vi "connect.vi"(0 "username":string="user", 1 "schema":string="public", 5 "password":string="password", 7 "host":string="localhost", 9 "port":i32=33060, 11 "error in (no error)":errorcluster) -> (4 "DB Session ID":i32, 15 "error out":errorcluster)   [LabVIEW 2022 SP3, in "Database.lvlib"]
uses:
  Database.lvlib
  bin/Database.dll
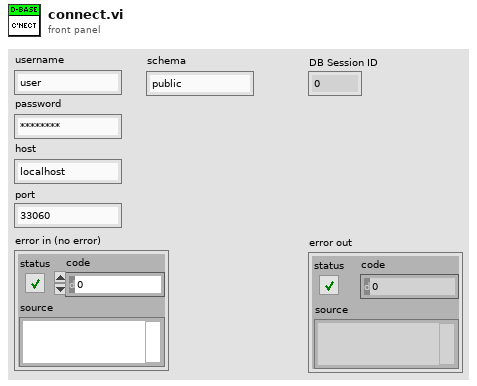
[diagram p1: front panel]
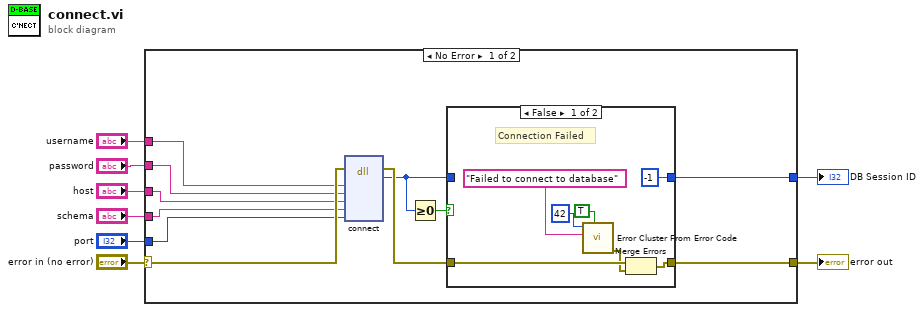
[diagram p0: block diagram]
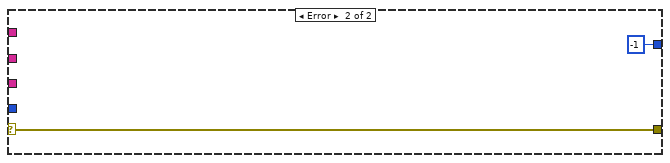
[diagram p3: hidden frame]
diagram:
  n1 = case shown="No Error" "error in (no error)" {
    selector: "error in (no error)" -> [w19 w30]
    tunnel: [w15 w30] -> w7
    tunnel: "username" -> [w13 _]
    tunnel: "password" -> [w12 _]
    tunnel: "host" -> [w11 _]
    tunnel: "port" -> [w10 _]
    tunnel: [w14 -1 ("return type")] -> w2
    tunnel: "schema" -> [w9 _]
    frame No Error {
      n2 = dll-call lib="C:/Users/Caleb/Desktop/nebraska-silicon-lab/pixel-gantry-control/Gantry/Shared Components/bin/Database.dll" fn="connect"(error in=w19, "username"=w13, "password"=w12, "url"=w11, "schema"=w9, "port"=w10) -> (error out=w17:errorcluster, "return type"=w16:i32)  [unwired: 7 in, 1 out]
      n3 = Greater Or Equal To 0?(x=w16) -> (x >= 0?=w18:bool)
      n4 = case shown="False" w18 {
        tunnel: w17 -> [w25 w27]
        tunnel: w16 -> [_ w28]
        tunnel: [-1 ("return type") w28] -> w14
        tunnel: [w24 w27] -> w15
        frame False {
          # "Connection Failed"
          n5 = call <vilib>:"Error Cluster From Error Code.vi"("show call chain? (False)"=TRUE, "error message (\"\")"="Failed to connect to database" ("error message (\"\")"), "error code (0)"=42) -> ("error out"=w23:errorcluster)  [unwired: 6 in]
          n6 = Merge Errors(w25, w23) -> (w24:errorcluster)
        }
        frame True {
          # "Connection Successful"
        }
      }
    }
    frame Error {
    }
  }
  "error out" <- w7
  "DB Session ID" <- w2
